vi "TestCompleteData.vi"(5 "Mode1":bool, 10 "ProductID":string, 11 "MES":T1) -> (2 "TestComplete in":T2)   [LabVIEW 2017]
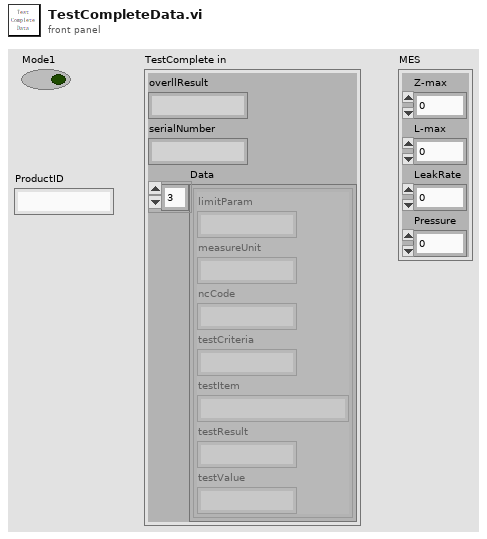
[diagram p1: front panel]
types:
  T1 = cluster{"Z-max":dbl, "L-max":dbl, "LeakRate":dbl, "Pressure":dbl}
  T2 = cluster{"overllResult":string, "serialNumber":string, "Data":cluster{"limitParam":string, "measureUnit":string, "ncCode":string, "testCriteria":string, "testItem":string, "testResult":string, "testValue":string}[]}
  T3 = cluster{"limitParam":string, "measureUnit":string, "ncCode":string, "testCriteria":string, "testItem":string, "testResult":string, "testValue":string}
  T4 = typedef "HD Config.ctl" = cluster{"ConnectPLC":cluster{"PLC Address":u8[], "PLC Port":i32, "PC Address":u8[]}, "FCO Model 4":cluster{"Com":refnum<visa-resource-name>, "Port":u32}, "FCO Model 7":cluster{"Com":refnum<visa-resource-name>, "Port":u32}, "Flow meter":cluster{"Com":refnum<visa-resource-name>, "Port":u32, "Units":enum16{"Standard", "Volumetric"}}}
  T5 = cluster{"limitParam":string, "measureUnit":string, "ncCode":string, "testCriteria":string, "testItem":string, "testResult":string, "testValue":string}[]
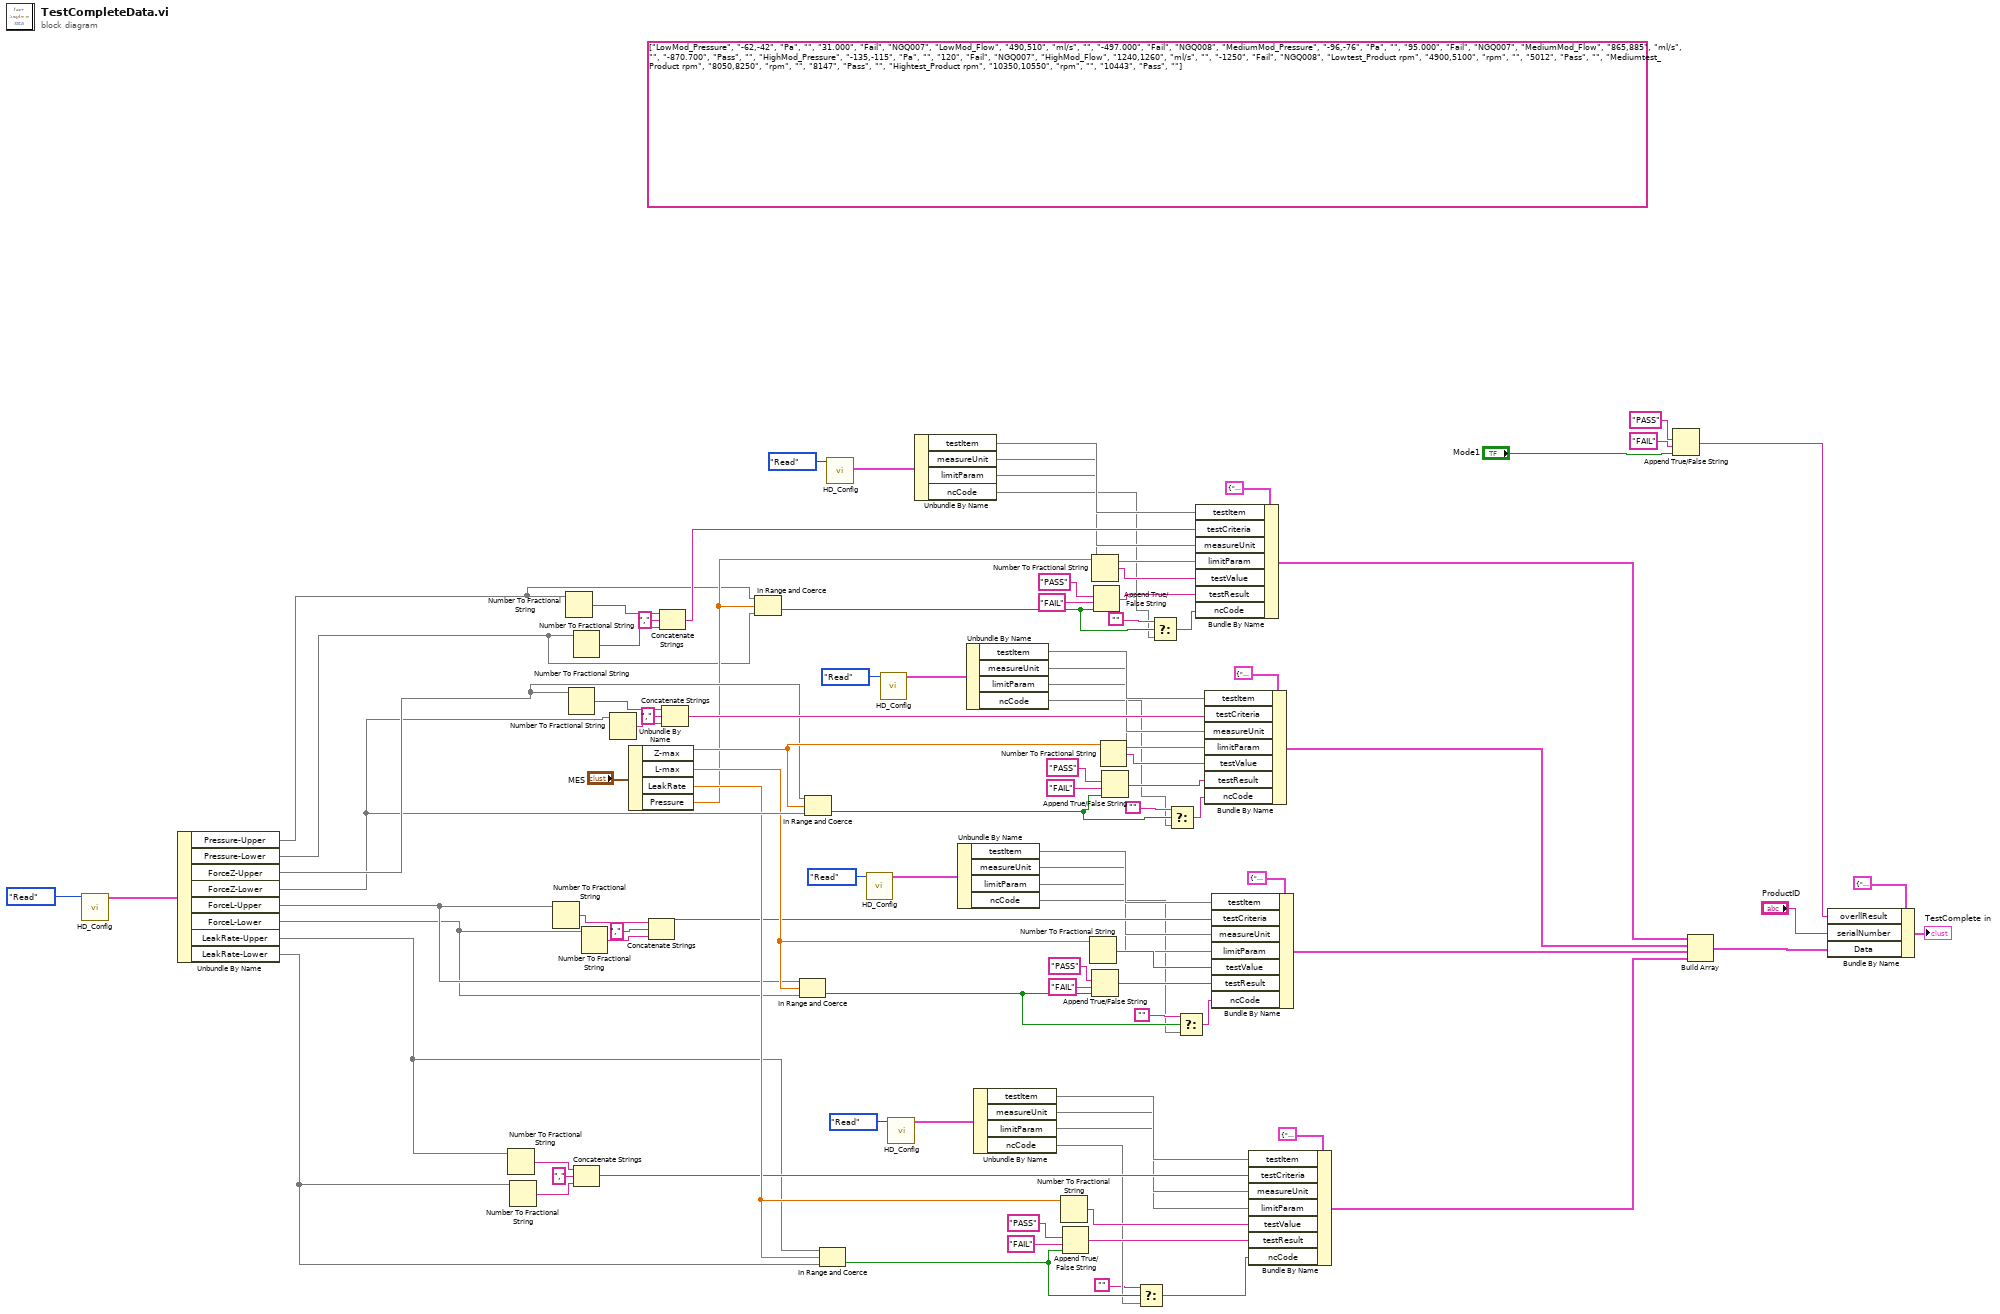
[diagram p0: block diagram]
diagram:
  (unwired) string[][] [["LowMod_Pressure", "-62,-42", "Pa", "", "31.000", "Fail", "NGQ007"], ["LowMod_Flow", "490,510", "ml/s", "", "-497.000", "Fail", "NGQ008"], ["MediumMod_Pressure", "-96,-76", "Pa", "", "95.000", "Fail", "NGQ007"], ["MediumMod_Flow", "865,885", "ml/s", "", "-870.700", "Pass", ""], ["HighMod_Pressure", "-135,-115", "Pa", "", "120", "Fail", "NGQ007"], ["HighMod_Flow", "1240,1260", "ml/s", "", "-1250", "Fail", "NGQ008"], ["Lowtest_Product rpm", "4900,5100", "rpm", "", "5012", "Pass", ""], ["Mediumtest_Product rpm", "8050,8250", "rpm", "", "8147", "Pass", ""], ["Hightest_Product rpm", "10350,10550", "rpm", "", "10443", "Pass", ""]] ("Testitems List Out")
  n1 = call "HD_Config.vi"("Step"=enum16{"Initial", "Write", "Read"}."Read") -> ("HD Config out"=w58:T4)  [unwired: 9 in, 1 out]
  n2 = Unbundle By Name(w58) -> ("Pressure-Upper"=w40, "Pressure-Lower"=w39, "ForceZ-Upper"=w63, "ForceZ-Lower"=w62, "ForceL-Upper"=w55, "ForceL-Lower"=w54, "LeakRate-Upper"=w53, "LeakRate-Lower"=w52)
  n3 = Number To Fractional String(number=w53) -> (F-format string=w84:string)  [unwired: 3 in]
  n4 = Number To Fractional String(number=w52) -> (F-format string=w83:string)  [unwired: 3 in]
  n5 = Number To Fractional String(number=w55) -> (F-format string=w81:string)  [unwired: 3 in]
  n6 = Number To Fractional String(number=w40) -> (F-format string=w44:string)  [unwired: 3 in]
  n7 = Number To Fractional String(number=w63) -> (F-format string=w87:string)  [unwired: 3 in]
  n8 = Number To Fractional String(number=w39) -> (F-format string=w43:string)  [unwired: 3 in]
  n9 = Concatenate Strings(w84, "," ("字符串"), w83) -> (w57:string)
  n10 = Number To Fractional String(number=w54) -> (F-format string=w80:string)  [unwired: 3 in]
  n11 = Number To Fractional String(number=w62) -> (F-format string=w88:string)  [unwired: 3 in]
  n12 = Unbundle By Name("MES") -> ("Z-max"=w64:dbl, "L-max"=w61:dbl, "LeakRate"=w60:dbl, "Pressure"=w41:dbl)
  n13 = Concatenate Strings(w81, "," ("字符串"), w80) -> (w56:string)
  n14 = Concatenate Strings(w44, "," ("字符串"), w43) -> (w42:string)
  n15 = Concatenate Strings(w87, "," ("字符串"), w88) -> (w65:string)
  n16 = In Range and Coerce(upper limit=w40, x=w41, lower limit=w39) -> (In Range?=w3:bool)  [unwired: 1 out]
  n17 = In Range and Coerce(upper limit=w55, x=w61, lower limit=w54) -> (In Range?=w11:bool)  [unwired: 1 out]
  n18 = In Range and Coerce(upper limit=w63, x=w64, lower limit=w62) -> (In Range?=w7:bool)  [unwired: 1 out]
  n19 = In Range and Coerce(upper limit=w53, x=w60, lower limit=w52) -> (In Range?=w16:bool)  [unwired: 1 out]
  n20 = call "HD_Config.vi"("Step"=enum16{"Initial", "Write", "Read"}."Read") -> ("HD Config out"=w35:T4)  [unwired: 9 in, 1 out]
  n21 = call "HD_Config.vi"("Step"=enum16{"Initial", "Write", "Read"}."Read") -> ("HD Config out"=w25:T4)  [unwired: 9 in, 1 out]
  n22 = call "HD_Config.vi"("Step"=enum16{"Initial", "Write", "Read"}."Read") -> ("HD Config out"=w30:T4)  [unwired: 9 in, 1 out]
  n23 = call "HD_Config.vi"("Step"=enum16{"Initial", "Write", "Read"}."Read") -> ("HD Config out"=w20:T4)  [unwired: 9 in, 1 out]
  n24 = Unbundle By Name(w35) -> ("testItem"=w34, "measureUnit"=w33, "limitParam"=w32, "ncCode"=w2)
  n25 = Unbundle By Name(w25) -> ("testItem"=w24, "measureUnit"=w23, "limitParam"=w22, "ncCode"=w10)
  n26 = Unbundle By Name(w30) -> ("testItem"=w29, "measureUnit"=w28, "limitParam"=w27, "ncCode"=w6)
  n27 = Unbundle By Name(w20) -> ("testItem"=w19, "measureUnit"=w18, "limitParam"=w17, "ncCode"=w15)
  n28 = Number To Fractional String(number=w60) -> (F-format string=w70:string)  [unwired: 3 in]
  n29 = Append True/False String(1:w16, 2:"FAIL", 3:"PASS") -> (0:w71:string)  [unwired: 1 in]
  n30 = Number To Fractional String(number=w61) -> (F-format string=w74:string)  [unwired: 3 in]
  n31 = Number To Fractional String(number=w41) -> (F-format string=w48:string)  [unwired: 3 in]
  n32 = Append True/False String(1:w11, 2:"FAIL", 3:"PASS") -> (0:w73:string)  [unwired: 1 in]
  n33 = Append True/False String(1:w3, 2:"FAIL", 3:"PASS") -> (0:w49:string)  [unwired: 1 in]
  n34 = Number To Fractional String(number=w64) -> (F-format string=w79:string)  [unwired: 3 in]
  n35 = Append True/False String(1:w7, 2:"FAIL", 3:"PASS") -> (0:w78:string)  [unwired: 1 in]
  n36 = Select(t="", s=w16, f=w15) -> (s? t:f=w13:string)
  n37 = Select(t="", s=w3, f=w2) -> (s? t:f=w1:string)
  n38 = Select(t="", s=w7, f=w6) -> (s? t:f=w5:string)
  n39 = Select(t="", s=w11, f=w10) -> (s? t:f=w9:string)
  n40 = Bundle By Name(cluster=T3 {"limitParam"="", "measureUnit"="", "ncCode"="", "testCriteria"="", "testItem"="", "testResult"="", "testValue"=""} ("Model1Data1"), "testItem"=w34, "testCriteria"=w42, "measureUnit"=w33, "limitParam"=w32, "testValue"=w48, "testResult"=w49, "ncCode"=w1) -> (w38:T3)
  n41 = Bundle By Name(cluster=T3 {"limitParam"="", "measureUnit"="", "ncCode"="", "testCriteria"="", "testItem"="", "testResult"="", "testValue"=""} ("Model1Data1"), "testItem"=w29, "testCriteria"=w65, "measureUnit"=w28, "limitParam"=w27, "testValue"=w79, "testResult"=w78, "ncCode"=w5) -> (w92:T3)
  n42 = Bundle By Name(cluster=T3 {"limitParam"="", "measureUnit"="", "ncCode"="", "testCriteria"="", "testItem"="", "testResult"="", "testValue"=""} ("Model1Data1"), "testItem"=w24, "testCriteria"=w56, "measureUnit"=w23, "limitParam"=w22, "testValue"=w74, "testResult"=w73, "ncCode"=w9) -> (w72:T3)
  n43 = Bundle By Name(cluster=T3 {"limitParam"="", "measureUnit"="", "ncCode"="", "testCriteria"="", "testItem"="", "testResult"="", "testValue"=""} ("Model1Data1"), "testItem"=w19, "testCriteria"=w57, "measureUnit"=w18, "limitParam"=w17, "testValue"=w70, "testResult"=w71, "ncCode"=w13) -> (w66:T3)
  n44 = Append True/False String(1:"Mode1", 2:"FAIL", 3:"PASS") -> (0:w95:string)  [unwired: 1 in]
  n45 = Build Array(w38, w92, w72, w66) -> (w93:T5)
  n46 = Bundle By Name(cluster=T2 {"overllResult"="", "serialNumber"="", "Data"=[]} ("TestComplete in"), "overllResult"=w95, "serialNumber"="ProductID", "Data"=w93) -> (→"TestComplete in":T2)
